vi "Base command.vi"(0 "Marca":T2, 5 "Comando":T1, 7 "Parametro 1":string, 9 "Parametro 2":string, 11 "error in (no error)":errorcluster) -> (6 "Command":string, 15 "error out":errorcluster)   [LabVIEW 2019, in "Serial Device.lvclass"]
uses:
  Serial Device.lvclass
  Marca.ctl
  Comando.ctl
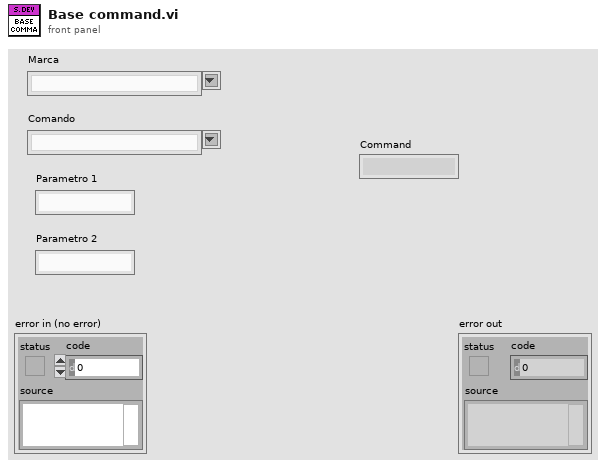
[diagram p1: front panel]
types:
  T1 = typedef "Comando.ctl" = string
  T2 = typedef "Marca.ctl" = string
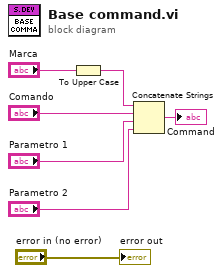
[diagram p0: block diagram]
diagram:
  n1 = To Upper Case(1:"Marca") -> (0:w3:T2)
  n2 = Concatenate Strings(w3, "Comando", "Parametro 1", "Parametro 2") -> (→"Command":string)
  "error out" <- "error in (no error)"
